vi "Set File For Save.vi"(8 "error in (no error)":errorcluster caption="entrée d'erreur (pas d'erreur)", 10 "File For Save":refnum<queue>, 11 "Class Log_File (Default) en entrée":refnum<class "Class Log_File (Default).lvclass">) -> (0 "error out":errorcluster caption="sortie d'erreur", 3 "Class Log_File (Default) en sortie":refnum<class "Class Log_File (Default).lvclass">)   [LabVIEW 2020, in "Library Instrument & Equipement.lvlib" / "Library Log_File.lvlib" / "Class Log_File (Default).lvclass"]
uses:
  Class Log_File (Default).lvclass
  Commun VI/TypeDef/Commande Test/Commande Data Test.ctl
  Commun VI/TypeDef/Commande Test/Commande Value Type.ctl
  Commun VI/TypeDef/Commande Test/Commande Type Test.ctl
  Class Log_File (Default).lvclass/Class Log_File (Default).ctl
  Commun VI/Library Commun.lvlib
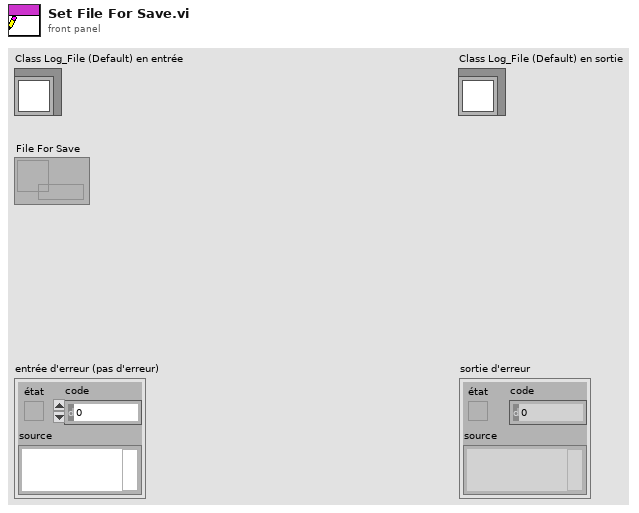
[diagram p1: front panel]
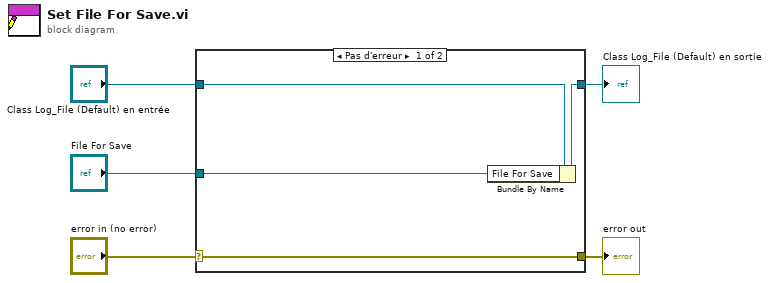
[diagram p0: block diagram]
diagram:
  n1 = case shown="Pas d'erreur" "error in (no error)" {
    selector: "error in (no error)" -> [w9 w10]
    tunnel: [w9 w10] -> w4
    tunnel: [w7 w11] -> w2
    tunnel: "Class Log_File (Default) en entrée" -> [w8 w11]
    tunnel: "File For Save" -> [w6 _]
    frame No Error {
      n2 = Bundle By Name(cluster=w8, "File For Save"=w6) -> (w7:refnum<class "Class Log_File (Default).lvclass">)
    }
    frame Error {
    }
  }
  "error out" <- w4
  "Class Log_File (Default) en sortie" <- w2
